vi "Split Registers by Direction.vi"(7 "Group":bool, 8 "error in":errorcluster, 11 "vi info":T1 {"RegisterMap"."Address" format="%.0x"}) -> (0 "error out":errorcluster, 2 "Controls":T8[](array[typedef]) {"Data Type" format="%.0x"}, 3 "Indicator":T8[](array[typedef]) {"Data Type" format="%.0x"})   [LabVIEW 2026, in "FPGA Addon System Explorer.lvlib"]
uses:
  FPGA Addon System Explorer.lvlib
  <userlib>/_OpenG.lib/lvdata/lvdata.llb/openg_variant.lvlib
  Addon Shared/Types/Register Information.ctl
  Addon Shared/FPGA Addon Shared.lvlib
  Submodules/Source/Types/PWM.Measure.Analog.Measurement.ctl
  Submodules/Source/Speciality FPGA IO.lvlib
  Addon Shared/Types/FPGA Addon Data Type.ctl
  Submodules/Source/Types/PWM.Measure.Digital.Measurement.ctl
  Submodules/Source/Types/PWM.Generate.Digital.Settings.ctl
  Submodules/Source/Types/PWM.Measure.Analog.Settings.ctl
  Submodules/Source/Types/PWM.Measure.Digital.Settings.ctl
  Submodules/Source/Types/Sine.Generate.Settings.ctl
  Submodules/Source/Types/Static.Measure.Digital.Measurement.ctl
  Submodules/Source/Types/Static.Generate.Digital.Settings.ctl
  Submodules/Source/Types/Static.Measure.Digital.Settings.ctl
  Submodules/Source/Types/WSS.Generate.Digital.Settings.ctl
  Submodules/Source/Types/QuadratureEncoder.Measure.Digital.Settings.ctl
  Submodules/Source/Types/QuadratureEncoder.Measure.Digital.Measurement.ctl
  <vilib>/fxp/LVFixedPointRepRangeTypeDef.ctl
  <vilib>/fxp/LVFixedPointRepBitsTypeDef.ctl
  <vilib>/Utility/Data Type/NI_Data Type.lvlib
  APIs/FPGA Register IO/TypeDefs/FXP Configuration.ctl
  APIs/FPGA Register IO/FPGA Register IO.lvlib
  <vilib>/picture/picture.llb/imagedata.ctl
  <vilib>/rvi/Bitfile/nirviTypdefDescription.ctl
  <vilib>/rvi/Bitfile/nirviMechanicalAction.ctl
  <vilib>/rvi/Bitfile/nirviClusterElementControl.ctl
  <vilib>/rvi/Bitfile/nirviSubControlStructure.ctl
  <vilib>/rvi/Bitfile/nirviControlStructure.ctl
  <vilib>/rvi/Bitfile/niFpgaBitfileStructure_VI.ctl
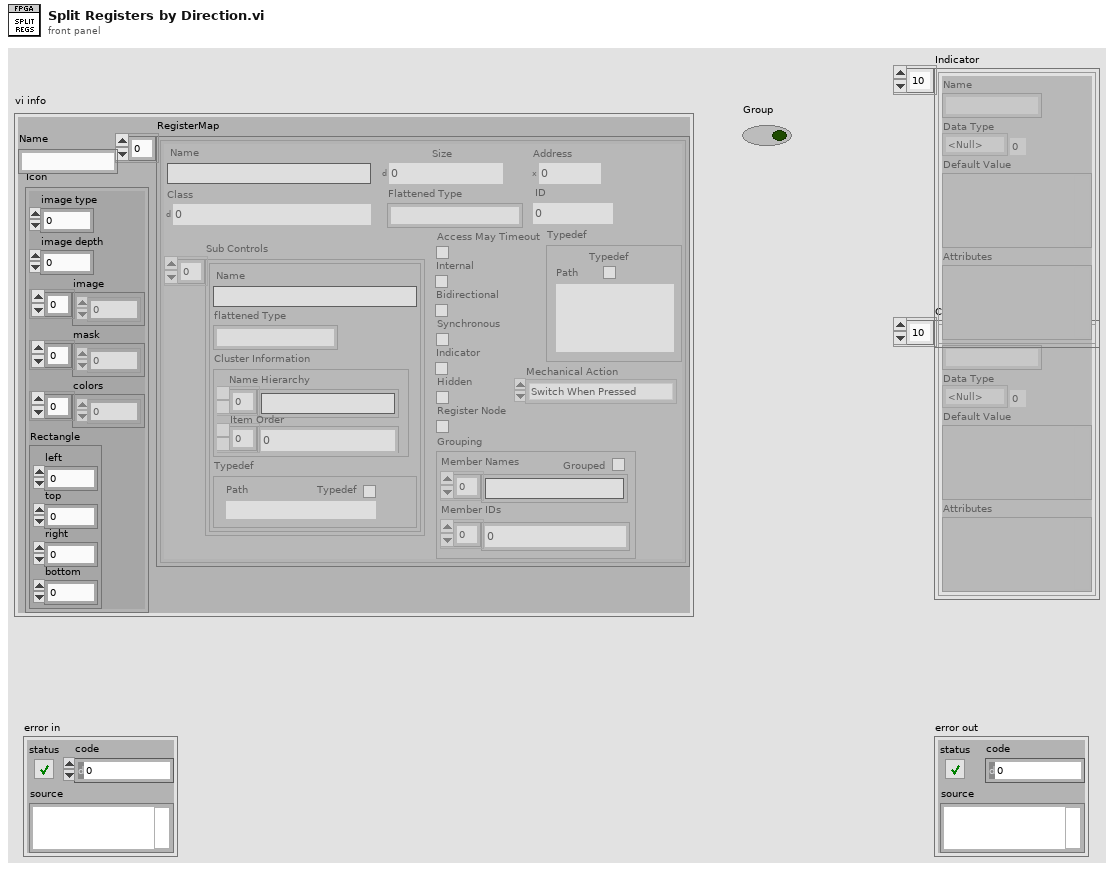
[diagram p1: front panel]
types:
  T1 = typedef "niFpgaBitfileStructure_VI.ctl" = cluster{"Name":string, "RegisterMap":T2[], "Icon":T7}
  T2 = typedef "nirviControlStructure.ctl" = cluster{"Name":string, "Hidden":bool, "Indicator":bool, "Flattened Type":string, "Grouping":cluster{"Grouped":bool, "Member Names":string[], "Member IDs":u32[]}, "Address":u32, "Size":u32, "Class":u32, "Internal":bool, "Typedef":T3, "ID":u32, "Bidirectional":bool, "Synchronous":bool, "Mechanical Action":T4, "Sub Controls":T5[], "Access May Timeout":bool, "Register Node":bool}
  T3 = typedef "nirviTypdefDescription.ctl" = cluster{"Typedef":bool, "Path":path}
  T4 = typedef "nirviMechanicalAction.ctl" = enum8{"Switch When Pressed", "Switch When Released", "Switch Until Released", "Latch When Pressed", "Latch When Released", "Latch Until Released"}
  T5 = typedef "nirviSubControlStructure.ctl" = cluster{"Name":string, "flattened Type":string, "Cluster Information":T6, "Typedef":T3}
  T6 = typedef "nirviClusterElementControl.ctl" = cluster{"Name Hierarchy":string[], "Item Order":u32[]}
  T7 = typedef "imagedata.ctl" = cluster{"image type":i32, "image depth":i32, "image":u8[], "mask":u8[], "colors":u32[], "Rectangle":cluster{"left":i16, "top":i16, "right":i16, "bottom":i16}}
  T8 = typedef "FPGA Addon Shared.lvlib/Register Information.ctl" = cluster{"Name":string, "Data Type":T9, "Default Value":variant, "Attributes":variant}
  T9 = typedef "FPGA Addon Shared.lvlib/FPGA Addon Data Type.ctl" = enum8{"<Null>", "I8", "I16", "I32", "I64", "U8", "U16", "U32", "U64", "SGL", "Boolean", "Analog PWM In Settings", "Analog PWM In", "Digital PWM In Settings", "Digital PWM In", "Digital PWM Out", "Sine Out", "FXP", "FXP+/-24.5", "FXP+/-16.5", "FXP+/-32.8", "FXP+/-64.32", "FXP+/-16.7", "FXP+/-20.5", "FXP+/-27.5", "FXP+/-32.16", "FXP+16.3", "FXP+18.3", "Digital Static In", "Digital Static Out", "Digital Static In Settings", "Digital WSS Out", "Quad Encoder Settings", "Quad Encoder In", "Group"}
  T10 = typedef "Speciality FPGA IO.lvlib/QuadratureEncoder.Measure.Digital.Measurement.ctl" = cluster{"POSITION":i32}
  T11 = typedef "Speciality FPGA IO.lvlib/Static.Measure.Digital.Measurement.ctl" = cluster{"STATE":bool}
  T12 = typedef "Speciality FPGA IO.lvlib/PWM.Measure.Digital.Measurement.ctl" = cluster{"ACTIVE TICKS":u32, "INACTIVE TICKS":u32, "ACQ TICKS":u32}
  T13 = typedef "Speciality FPGA IO.lvlib/PWM.Measure.Analog.Measurement.ctl" = cluster{"ACTIVE TICKS":u32, "INACTIVE TICKS":u32, "ACQ TICKS":u32, "ACTIVE VOLTAGE":fxp<+/-,32,8>, "INACTIVE VOLTAGE":fxp<+/-,32,8>}
  T14 = typedef "Speciality FPGA IO.lvlib/QuadratureEncoder.Measure.Digital.Settings.ctl" = cluster{"DIRECTION":u8, "RESET VALUE":i32, "A RESET STATE":bool, "B RESET STATE":bool, "Z RESET STATE":bool}
  T15 = typedef "Speciality FPGA IO.lvlib/WSS.Generate.Digital.Settings.ctl" = cluster{"ACTIVE EDGE":bool, "ACTIVE TICKS":u32, "INACTIVE TICKS":u32, "DATA":u8, "SENSOR TYPE":u8}
  T16 = typedef "Speciality FPGA IO.lvlib/Static.Measure.Digital.Settings.ctl" = cluster{"ACTIVE EDGE":bool}
  T17 = typedef "Speciality FPGA IO.lvlib/Static.Generate.Digital.Settings.ctl" = cluster{"ACTIVE EDGE":bool, "OUTPUT":bool}
  T18 = typedef "Speciality FPGA IO.lvlib/Sine.Generate.Settings.ctl" = cluster{"AMP":fxp<+/-,32,8>, "OFFSET":fxp<+/-,32,8>, "PERIODS/TICKS":fxp<+,32,0>}
  T19 = typedef "Speciality FPGA IO.lvlib/PWM.Measure.Digital.Settings.ctl" = cluster{"ACTIVE EDGE":bool, "TIMEOUT":u32}
  T20 = typedef "Speciality FPGA IO.lvlib/PWM.Measure.Analog.Settings.ctl" = cluster{"ACTIVE EDGE":bool, "TIMEOUT":u32, "THRESHOLD":fxp<+/-,32,8>}
  T21 = typedef "Speciality FPGA IO.lvlib/PWM.Generate.Digital.Settings.ctl" = cluster{"ACTIVE EDGE":bool, "ACTIVE TICKS":u32, "INACTIVE TICKS":u32}
  T22 = typedef "FPGA Register IO.lvlib/FXP Configuration.ctl" = cluster{"FXP Representation":T23, "FXP Range":T24}
  T23 = typedef "LVFixedPointRepBitsTypeDef.ctl" = cluster{"Signed":bool, "Word Length":u32, "Integer Word Length":i32}
  T24 = typedef "LVFixedPointRepRangeTypeDef.ctl" = cluster{"Range Min":dbl, "Range Max":dbl, "Delta":dbl}
  T25 = typedef "openg_variant.lvlib/Type Descriptor Enumeration__ogtk.ctl" = enum8{"<Null>", "I8", "I16", "I32", "I64", "U8", "U16", "U32", "U64", "SGL", "DBL", "EXT", "CSG", "CDB", "CXT", "0x0F", "0x10", "0x11", "0x12", "0x13", "0x14", "Enum U8", "Enum U16", "Enum U32", "Enum U64", "SGL PQ", "DBL PQ", "EXT PQ", "CSG PQ", "CDB PQ", "CXT PQ", "0x1F", "0x20", "Boolean", "0x22", "0x23", "0x24", "0x25", "0x26", "0x27", "0x28", "0x29", "0x2A", "0x2B", "0x2C", "0x2D", "0x2E", "0x2F", "String", "0x31", "Path", "Pict", "0x34", "0x35", "0x36", "DAQ", "0x38", "0x39", "0x3A", "0x3B", "0x3C", "0x3D", "0x3E", "0x3F", "Array", "0x41", "0x42", "0x43", "0x44", "0x45", "0x46", "0x47", "0x48", "0x49", "0x4A", "0x4B", "0x4C", "0x4D", "0x4E", "0x4F", "Cluster", "0x51", "0x52", "Variant", "Waveform", "0x55", "0x56", "0x57", "0x58", "0x59", "0x5A", "0x5B", "0x5C", "0x5D", "0x5E", "Fixed Point", "0x60", "0x61", "0x62", "0x63", "0x64", "0x65", "0x66", "0x67", "0x68", "0x69", "0x6A", "0x6B", "0x6C", "0x6D", "0x6E", "0x6F", "Refnum", "0x71", "0x72", "Set Collection", "Map Collection"}
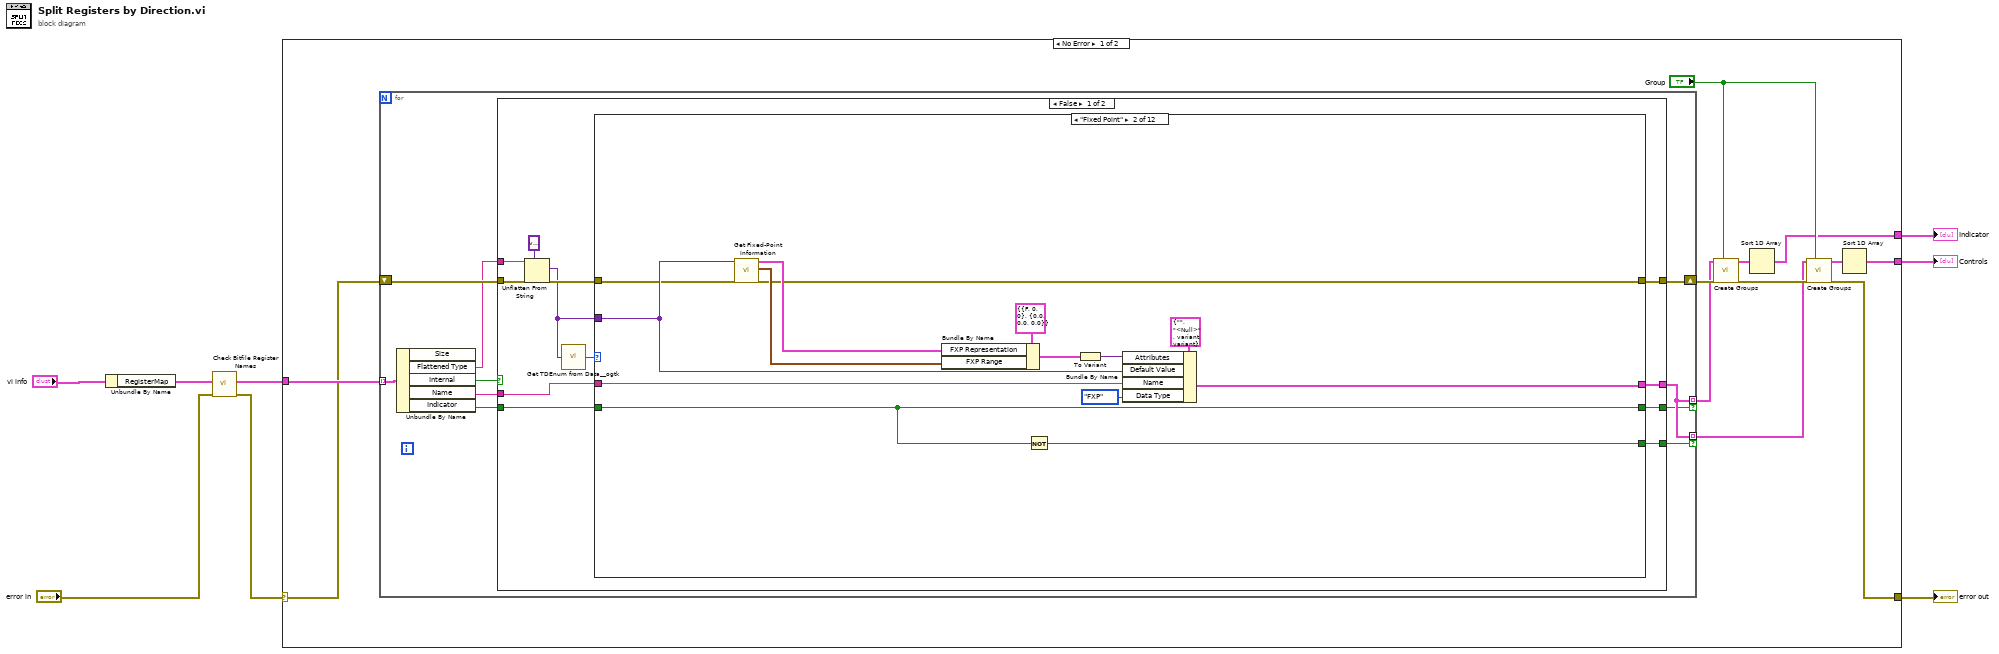
[diagram p0: block diagram]
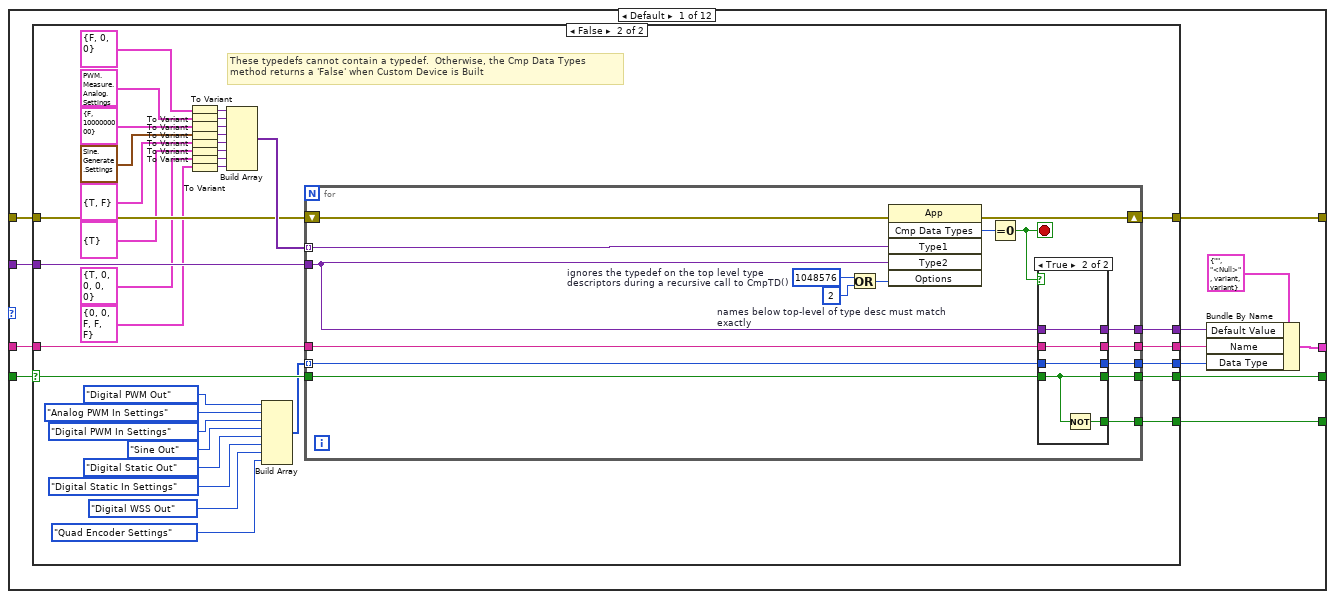
[diagram p2: hidden frame]
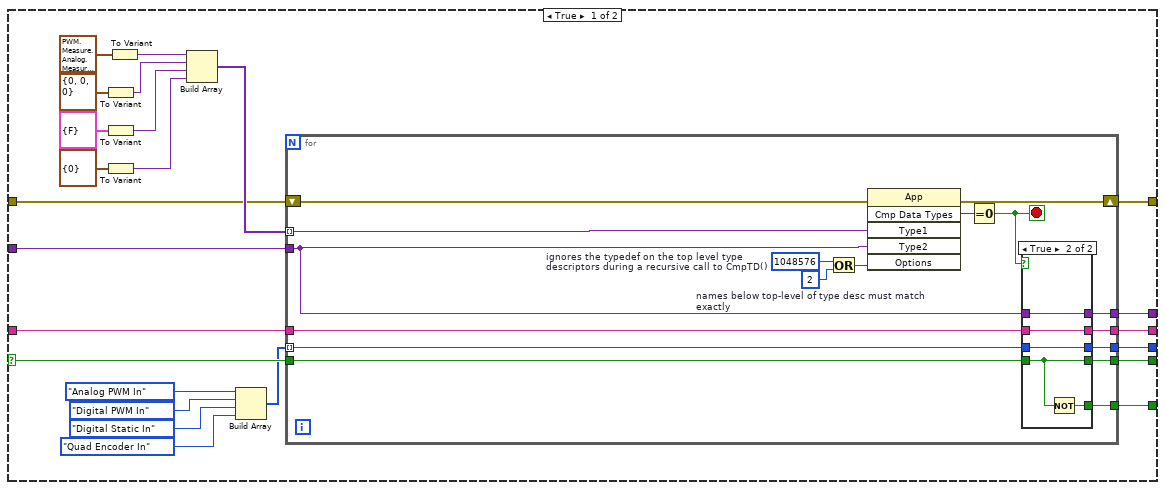
[diagram p3: hidden frame]
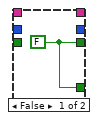
[diagram p4: hidden frame]
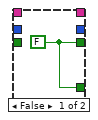
[diagram p5: hidden frame]
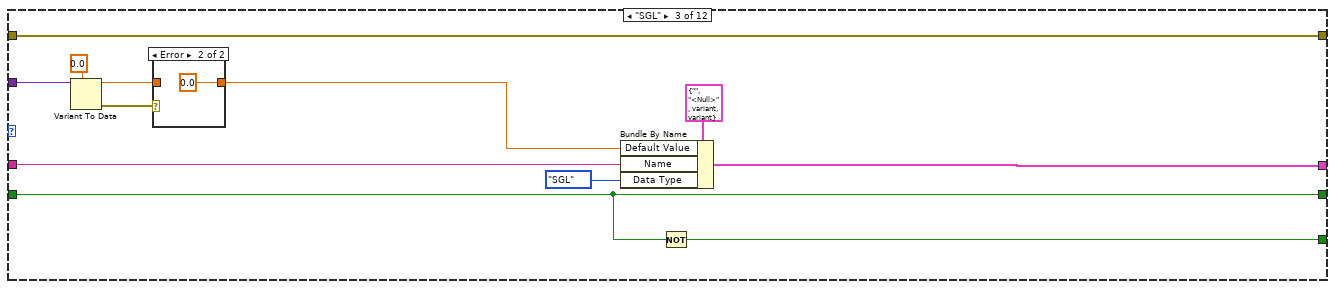
[diagram p6: hidden frame]
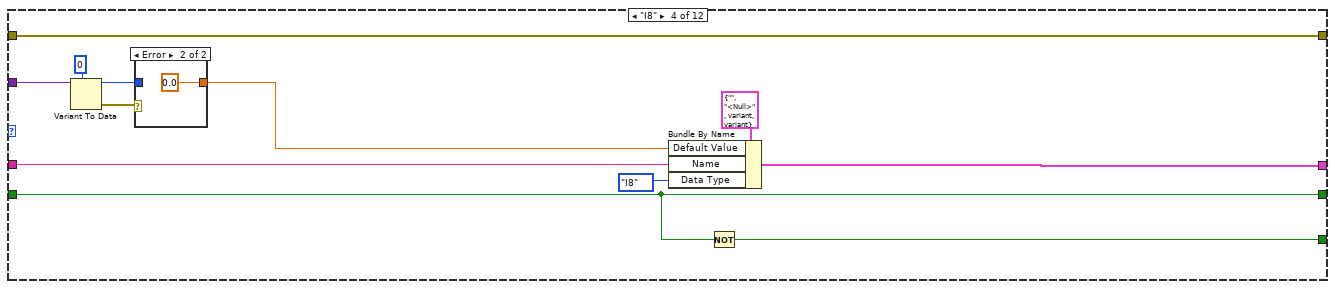
[diagram p8: hidden frame]
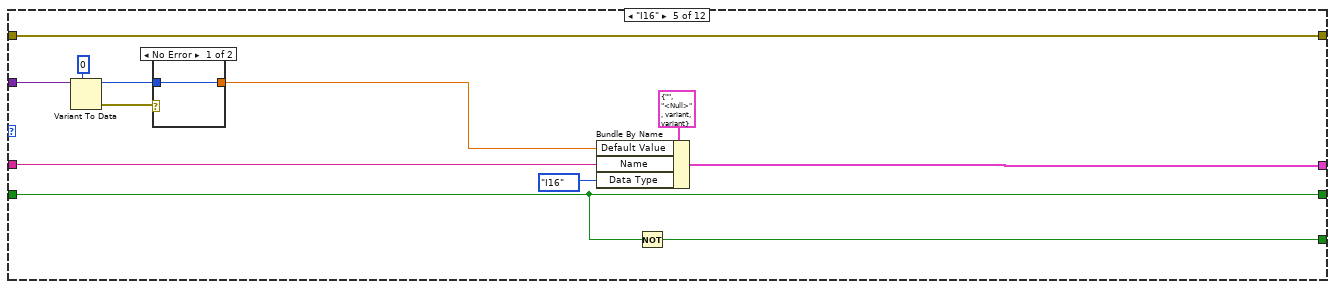
[diagram p10: hidden frame]
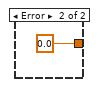
[diagram p11: hidden frame]
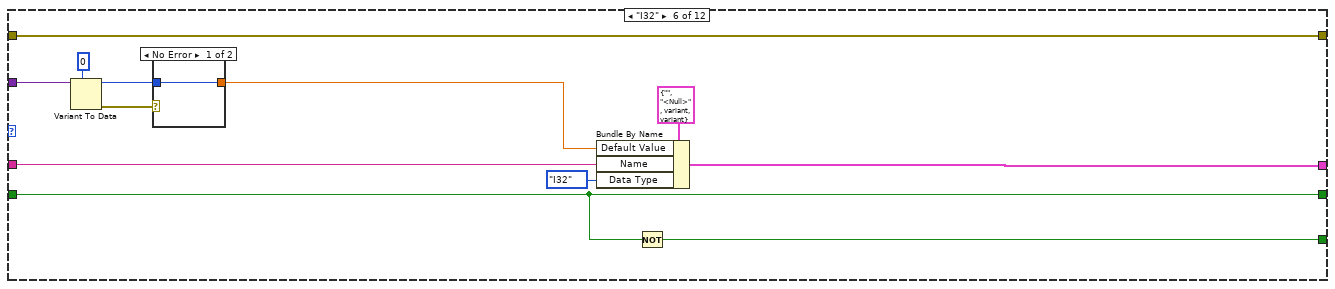
[diagram p12: hidden frame]
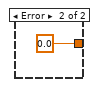
[diagram p13: hidden frame]
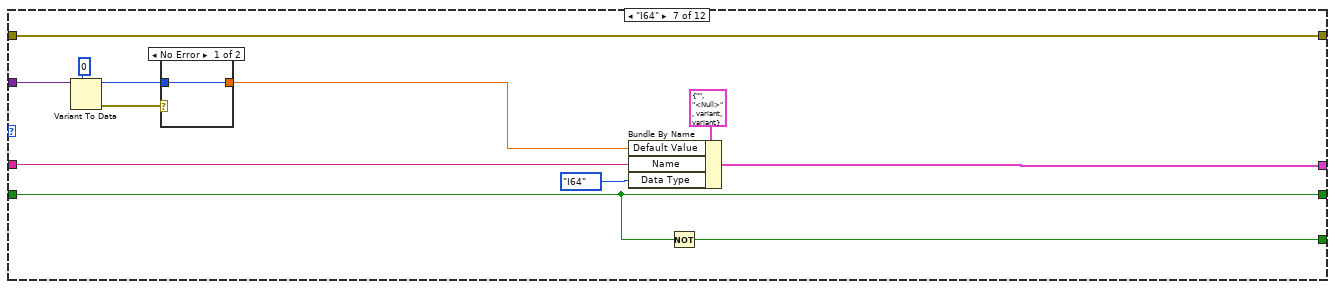
[diagram p14: hidden frame]
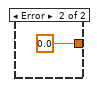
[diagram p15: hidden frame]
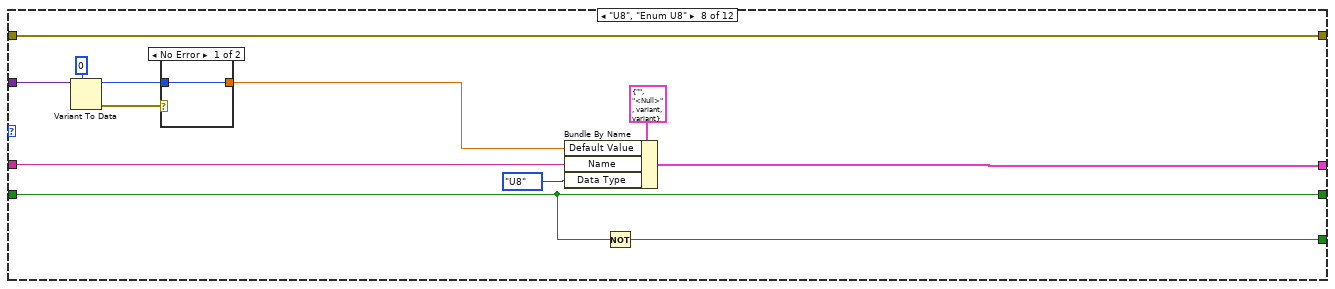
[diagram p16: hidden frame]
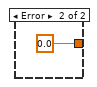
[diagram p17: hidden frame]
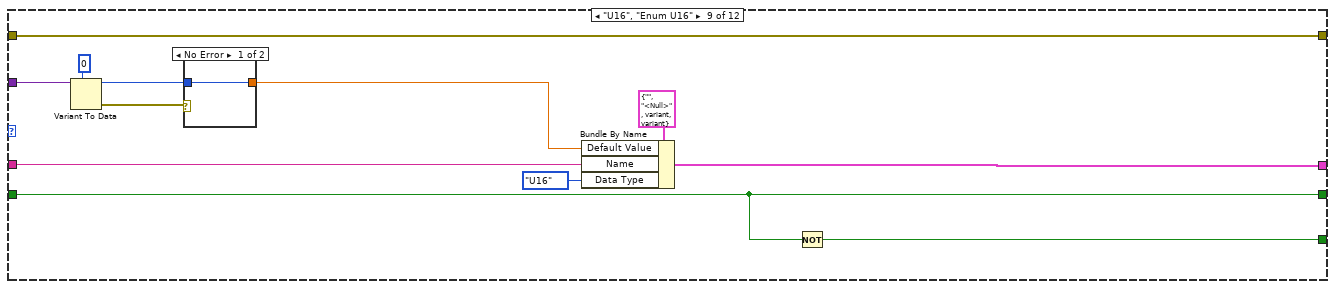
[diagram p18: hidden frame]
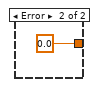
[diagram p19: hidden frame]
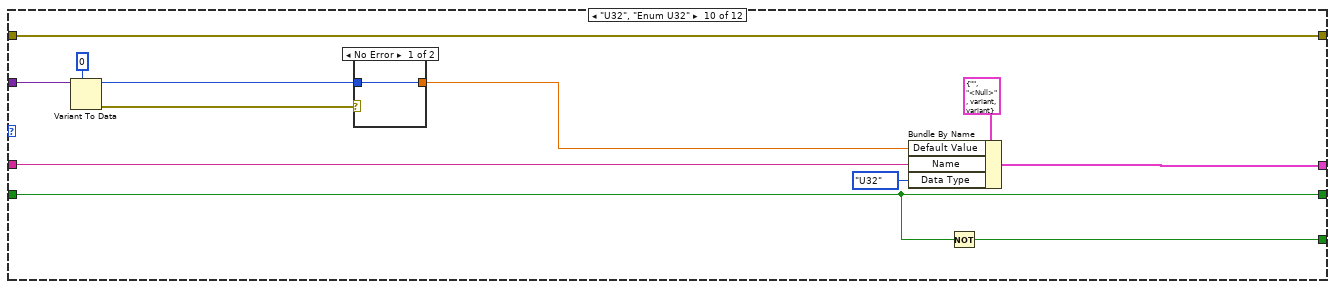
[diagram p20: hidden frame]
diagram:
  n1 = Unbundle By Name("vi info") -> ("RegisterMap"=w4:T2[])
  n2 = call "Check Bitfile Register Names.vi"("error in (no error)"="error in", "RegisterMap in"=w4) -> ("error out"=w1:errorcluster, "RegisterMap out"=w3:T2[])  [unwired: 8 in]
  n3 = case shown="No Error" w1 {
    selector: w1 -> [w9 w318]
    tunnel: [w18 w318] -> w7
    tunnel: [w13 _] -> w6
    tunnel: [w11 _] -> w5
    tunnel: w3 -> [w10 _]
    frame No Error {
      n4 = for {
        tunnel: w10 -> [w25] mode=indexing
        tunnel: [w30] -> w16 mode=indexing if=w29
        tunnel: [w30] -> w15 mode=indexing if=w28
        shift-right: [w27] -> w20
        shift-left: w9 -> [w26]
        n5 = Unbundle By Name(w25) -> ("Flattened Type"=w21:string, "Internal"=w22:bool, "Name"=w23:string, "Indicator"=w24:bool)  [unwired: 1 out]
        n6 = case shown="False" w22 {
          tunnel: w23 -> [w41 _]
          tunnel: w24 -> [w40 _]
          tunnel: [w39 _] -> w30
          tunnel: [w38 w317] -> w29
          tunnel: [w37 w317] -> w28
          tunnel: w21 -> [w34 _]
          tunnel: [w36 w316] -> w27
          tunnel: w26 -> [w33 w316]
          frame False {
            n7 = Unflatten From String(type=variant ("Variant"), binary string=w34, error in (no error)=w33) -> (value=w31:variant, error out=w32:errorcluster)  [unwired: 3 out]
            n8 = call <userlib>:"Get TDEnum from Data__ogtk.vi"("Data"=w31) -> ("Type Descriptor Enumeration"=w42:T25)  [unwired: 4 in]
            n9 = case shown="\"Fixed Point\"" w42 {
              tunnel: [w54 w174 w183 w197 w211 w225 w239 w253 w267 w281 w295 w309] -> w38
              tunnel: w40 -> [w49 w174 w183 w197 w211 w225 w239 w253 w267 w281 w295 w309]
              tunnel: w41 -> [w50 w170 w185 w199 w213 w227 w241 w255 w269 w283 w297 w311]
              tunnel: [w51 w171 w184 w198 w212 w226 w240 w254 w268 w282 w296 w310] -> w39
              tunnel: [w53 w173 w182 w196 w210 w224 w238 w252 w266 w280 w294 w308] -> w37
              tunnel: w31 -> [w48 w168 w181 w195 w209 w223 w237 w251 w265 w279 w293 w307]
              tunnel: [w44 w161 w175 w189 w203 w217 w231 w245 w259 w273 w287 w301] -> w36
              tunnel: w32 -> [w43 w167 w175 w189 w203 w217 w231 w245 w259 w273 w287 w301]
              frame Default {
                n10 = case shown="False" w49 {
                  selector: w49 -> [w73 w133]
                  tunnel: [w78 w137] -> w54
                  tunnel: [w77 w136] -> w53
                  tunnel: w50 -> [w76 w135]
                  tunnel: w48 -> [w67 w129]
                  tunnel: [w66 w128] -> w47
                  tunnel: [w65 w127] -> w46
                  tunnel: [w64 w126] -> w45
                  tunnel: [w62 w117] -> w44
                  tunnel: w43 -> [w61 w118]
                  frame True {
                    n11 = To Variant(anything=T12 {"ACTIVE TICKS"=0, "INACTIVE TICKS"=0, "ACQ TICKS"=0} ("Cached.Data")) -> (Variant=w71:variant)
                    n12 = To Variant(anything=T11 {"STATE"=FALSE} ("Cached.Data")) -> (Variant=w59:variant)
                    n13 = To Variant(anything=T10 {"POSITION"=0} ("Cached.Data")) -> (Variant=w55:variant)
                    n14 = To Variant(anything=T13 {"ACTIVE TICKS"=0, "INACTIVE TICKS"=0, "ACQ TICKS"=0, "ACTIVE VOLTAGE"=0.0, "INACTIVE VOLTAGE"=0.0} ("Cached.Data")) -> (Variant=w72:variant)
                    n15 = Build Array(w72, w71, w59, w55) -> (w68:variant[])
                    n16 = Build Array(FPGA_Addon_Data_Type."Analog PWM In" ("Data Type"), FPGA_Addon_Data_Type."Digital PWM In" ("Data Type"), FPGA_Addon_Data_Type."Digital Static In" ("Data Type"), FPGA_Addon_Data_Type."Quad Encoder In" ("Data Type")) -> (w63:T9[])
                    n17 = for {
                      tunnel: w67 -> [w82]
                      tunnel: [w93] -> w77
                      tunnel: w76 -> [w92]
                      tunnel: w68 -> [w84] mode=indexing
                      tunnel: [w91] -> w65
                      tunnel: [w90] -> w66
                      tunnel: [w89] -> w64
                      tunnel: w63 -> [w88] mode=indexing
                      tunnel: w73 -> [w95]
                      tunnel: [w94] -> w78
                      shift-right: [w79] -> w62
                      shift-left: w61 -> [w80]
                      stop <- w83 stop-if-true
                      w81 = 2  # names below top-level of type desc must match exactly
                      w86 = 1048576  # ignores the typedef on the top level type descriptors during a recursive call to CmpTD()
                      n18 = Or(x=w86, y=w81) -> (x .or. y?=w87:i32)
                      n19 = invoke class="App" method="Cmp Data Types"(error in=w80, "Type1"=w84, "Type2"=w82, "Options"=w87) -> (error out=w79:errorcluster, "Compare Data Types"=w85:i32)  [unwired: 2 in, 4 out]
                      n20 = Equal To 0?(x=w85) -> (x = 0?=w83:bool)
                      n21 = case shown="True" w83 {
                        tunnel: w95 -> [_ w101]
                        tunnel: [w96 w101] -> w94
                        tunnel: [w96 w100] -> w93
                        tunnel: w92 -> [_ w98]
                        tunnel: [_ w99] -> w91
                        tunnel: w82 -> [_ w99]
                        tunnel: [_ w98] -> w90
                        tunnel: [_ w97] -> w89
                        tunnel: w88 -> [_ w97]
                        frame False {
                          w96 = FALSE ("Boolean")
                        }
                        frame True {
                          n22 = Not(x=w101) -> (.not. x?=w100:bool)
                        }
                      }
                    }
                  }
                  frame False {
                    # "These typedefs cannot contain a typedef.  Otherwise, the Cmp Data Types \nmethod returns a 'False' when Custom Device is Built"
                    n23 = To Variant(anything=T21 {"ACTIVE EDGE"=FALSE, "ACTIVE TICKS"=0, "INACTIVE TICKS"=0} ("Channel.Settings")) -> (Variant=w132:variant)
                    n24 = To Variant(anything=T20 {"ACTIVE EDGE"=FALSE, "TIMEOUT"=1000000000, "THRESHOLD"=3.0} ("Channel.Settings")) -> (Variant=w122:variant)
                    n25 = To Variant(anything=T19 {"ACTIVE EDGE"=FALSE, "TIMEOUT"=1000000000} ("Channel.Settings")) -> (Variant=w121:variant)
                    n26 = To Variant(anything=T18 {"AMP"=0.0, "OFFSET"=0.0, "PERIODS/TICKS"=0.0002500000409781933} ("Settings")) -> (Variant=w115:variant)
                    n27 = To Variant(anything=T17 {"ACTIVE EDGE"=TRUE, "OUTPUT"=FALSE} ("Settings")) -> (Variant=w113:variant)
                    n28 = To Variant(anything=T16 {"ACTIVE EDGE"=TRUE} ("Settings")) -> (Variant=w110:variant)
                    n29 = To Variant(anything=T15 {"ACTIVE EDGE"=TRUE, "ACTIVE TICKS"=0, "INACTIVE TICKS"=0, "DATA"=0, "SENSOR TYPE"=0} ("Wheel Speed Sensor Settings")) -> (Variant=w106:variant)
                    n30 = To Variant(anything=T14 {"DIRECTION"=0, "RESET VALUE"=0, "A RESET STATE"=FALSE, "B RESET STATE"=FALSE, "Z RESET STATE"=FALSE} ("Settings")) -> (Variant=w103:variant)
                    n31 = Build Array(w132, w122, w121, w115, w113, w110, w106, w103) -> (w130:variant[])
                    n32 = Build Array(FPGA_Addon_Data_Type."Digital PWM Out" ("Data Type"), FPGA_Addon_Data_Type."Analog PWM In Settings" ("Data Type"), FPGA_Addon_Data_Type."Digital PWM In Settings" ("Data Type"), FPGA_Addon_Data_Type."Sine Out" ("Data Type"), FPGA_Addon_Data_Type."Digital Static Out" ("Data Type"), FPGA_Addon_Data_Type."Digital Static In Settings" ("Data Type"), FPGA_Addon_Data_Type."Digital WSS Out" ("Data Type"), FPGA_Addon_Data_Type."Quad Encoder Settings" ("Data Type")) -> (w125:T9[])
                    n33 = for {
                      tunnel: w129 -> [w143]
                      tunnel: [w152] -> w136
                      tunnel: w135 -> [w151]
                      tunnel: w130 -> [w142] mode=indexing
                      tunnel: [w150] -> w127
                      tunnel: [w149] -> w128
                      tunnel: [w148] -> w126
                      tunnel: w125 -> [w147] mode=indexing
                      tunnel: w133 -> [w154]
                      tunnel: [w153] -> w137
                      shift-right: [w138] -> w117
                      shift-left: w118 -> [w139]
                      stop <- w140 stop-if-true
                      w145 = 2  # names below top-level of type desc must match exactly
                      w144 = 1048576  # ignores the typedef on the top level type descriptors during a recursive call to CmpTD()
                      n34 = Or(x=w144, y=w145) -> (x .or. y?=w146:i32)
                      n35 = invoke class="App" method="Cmp Data Types"(error in=w139, "Type1"=w142, "Type2"=w143, "Options"=w146) -> (error out=w138:errorcluster, "Compare Data Types"=w141:i32)  [unwired: 2 in, 4 out]
                      n36 = Equal To 0?(x=w141) -> (x = 0?=w140:bool)
                      n37 = case shown="True" w140 {
                        tunnel: w154 -> [_ w160]
                        tunnel: [w155 w160] -> w153
                        tunnel: [w155 w159] -> w152
                        tunnel: w151 -> [_ w157]
                        tunnel: [_ w158] -> w150
                        tunnel: w143 -> [_ w158]
                        tunnel: [_ w157] -> w149
                        tunnel: [_ w156] -> w148
                        tunnel: w147 -> [_ w156]
                        frame False {
                          w155 = FALSE ("Boolean")
                        }
                        frame True {
                          n38 = Not(x=w160) -> (.not. x?=w159:bool)
                        }
                      }
                    }
                  }
                }
                n39 = Bundle By Name(cluster=T8 {"Name"="", "Data Type"=enum."<Null>", "Default Value"=variant(refnum<class> refnum), "Attributes"=variant}, "Default Value"=w46, "Name"=w47, "Data Type"=w45) -> (w51:T8)
              }
              frame "Fixed Point" {
                n40 = call <vilib>:"Get Fixed-Point Information.vi"("error in (no error)"=w167, "variant"=w168) -> ("error out"=w161:errorcluster, "FXP range"=w164:T24, "FXP representation"=w165:T23)  [unwired: 6 in, 1 out]
                n41 = Bundle By Name(cluster=T22 {"FXP Representation"={"Signed"=FALSE, "Word Length"=0, "Integer Word Length"=0}, "FXP Range"={"Range Min"=0.0, "Range Max"=0.0, "Delta"=0.0}} ("FXP Configuration"), "FXP Representation"=w165, "FXP Range"=w164) -> (w163:T22)
                n42 = Not(x=w174) -> (.not. x?=w173:bool)
                n43 = To Variant(anything=w163) -> (Variant=w162:variant)
                n44 = Bundle By Name(cluster=T8 {"Name"="", "Data Type"=enum."<Null>", "Default Value"=variant(refnum<class> refnum), "Attributes"=variant}, "Attributes"=w162, "Default Value"=w168, "Name"=w170, "Data Type"=FPGA_Addon_Data_Type."FXP") -> (w171:T8)
              }
              frame "SGL" {
                n45 = Variant To Data(type=sgl 0.0, Variant=w181) -> (data=w177:sgl, error out=w179:errorcluster)  [unwired: 1 in]
                n46 = case shown="Error" w179 {
                  tunnel: [w187 0.0] -> w178
                  tunnel: w177 -> [w187 _]
                  frame No Error {
                  }
                  frame Error {
                  }
                }
                n47 = Bundle By Name(cluster=T8 {"Name"="", "Data Type"=enum."<Null>", "Default Value"=variant(refnum<class> refnum), "Attributes"=variant}, "Default Value"=w178, "Name"=w185, "Data Type"=FPGA_Addon_Data_Type."SGL") -> (w184:T8)
                n48 = Not(x=w183) -> (.not. x?=w182:bool)
              }
              frame "I8" {
                n49 = Variant To Data(type=i8 0, Variant=w195) -> (data=w191:i8, error out=w193:errorcluster)  [unwired: 1 in]
                n50 = case shown="Error" w193 {
                  tunnel: [w201 0.0] -> w192
                  tunnel: w191 -> [w201 _]
                  frame No Error {
                  }
                  frame Error {
                  }
                }
                n51 = Bundle By Name(cluster=T8 {"Name"="", "Data Type"=enum."<Null>", "Default Value"=variant(refnum<class> refnum), "Attributes"=variant}, "Default Value"=w192, "Name"=w199, "Data Type"=FPGA_Addon_Data_Type."I8") -> (w198:T8)
                n52 = Not(x=w197) -> (.not. x?=w196:bool)
              }
              frame "I16" {
                n53 = Variant To Data(type=i16 0, Variant=w209) -> (data=w205:i16, error out=w207:errorcluster)  [unwired: 1 in]
                n54 = case shown="No Error" w207 {
                  tunnel: [w215 0.0] -> w206
                  tunnel: w205 -> [w215 _]
                  frame No Error {
                  }
                  frame Error {
                  }
                }
                n55 = Bundle By Name(cluster=T8 {"Name"="", "Data Type"=enum."<Null>", "Default Value"=variant(refnum<class> refnum), "Attributes"=variant}, "Default Value"=w206, "Name"=w213, "Data Type"=FPGA_Addon_Data_Type."I16") -> (w212:T8)
                n56 = Not(x=w211) -> (.not. x?=w210:bool)
              }
              frame "I32" {
                n57 = Variant To Data(type=0, Variant=w223) -> (data=w219:i32, error out=w221:errorcluster)  [unwired: 1 in]
                n58 = case shown="No Error" w221 {
                  tunnel: [w229 0.0] -> w220
                  tunnel: w219 -> [w229 _]
                  frame No Error {
                  }
                  frame Error {
                  }
                }
                n59 = Bundle By Name(cluster=T8 {"Name"="", "Data Type"=enum."<Null>", "Default Value"=variant(refnum<class> refnum), "Attributes"=variant}, "Default Value"=w220, "Name"=w227, "Data Type"=FPGA_Addon_Data_Type."I32") -> (w226:T8)
                n60 = Not(x=w225) -> (.not. x?=w224:bool)
              }
              frame "I64" {
                n61 = Variant To Data(type=i64 0, Variant=w237) -> (data=w233:i64, error out=w235:errorcluster)  [unwired: 1 in]
                n62 = case shown="No Error" w235 {
                  tunnel: [w243 0.0] -> w234
                  tunnel: w233 -> [w243 _]
                  frame No Error {
                  }
                  frame Error {
                  }
                }
                n63 = Bundle By Name(cluster=T8 {"Name"="", "Data Type"=enum."<Null>", "Default Value"=variant(refnum<class> refnum), "Attributes"=variant}, "Default Value"=w234, "Name"=w241, "Data Type"=FPGA_Addon_Data_Type."I64") -> (w240:T8)
                n64 = Not(x=w239) -> (.not. x?=w238:bool)
              }
              frame "U8", "Enum U8" {
                n65 = Variant To Data(type=u8 0, Variant=w251) -> (data=w247:u8, error out=w249:errorcluster)  [unwired: 1 in]
                n66 = case shown="No Error" w249 {
                  tunnel: [w257 0.0] -> w248
                  tunnel: w247 -> [w257 _]
                  frame No Error {
                  }
                  frame Error {
                  }
                }
                n67 = Bundle By Name(cluster=T8 {"Name"="", "Data Type"=enum."<Null>", "Default Value"=variant(refnum<class> refnum), "Attributes"=variant}, "Default Value"=w248, "Name"=w255, "Data Type"=FPGA_Addon_Data_Type."U8") -> (w254:T8)
                n68 = Not(x=w253) -> (.not. x?=w252:bool)
              }
              frame "U16", "Enum U16" {
                n69 = Variant To Data(type=u16 0, Variant=w265) -> (data=w261:u16, error out=w263:errorcluster)  [unwired: 1 in]
                n70 = case shown="No Error" w263 {
                  tunnel: [w271 0.0] -> w262
                  tunnel: w261 -> [w271 _]
                  frame No Error {
                  }
                  frame Error {
                  }
                }
                n71 = Bundle By Name(cluster=T8 {"Name"="", "Data Type"=enum."<Null>", "Default Value"=variant(refnum<class> refnum), "Attributes"=variant}, "Default Value"=w262, "Name"=w269, "Data Type"=FPGA_Addon_Data_Type."U16") -> (w268:T8)
                n72 = Not(x=w267) -> (.not. x?=w266:bool)
              }
              frame "U32", "Enum U32" {
                n73 = Variant To Data(type=u32 0, Variant=w279) -> (data=w275:u32, error out=w277:errorcluster)  [unwired: 1 in]
                n74 = case shown="No Error" w277 {
                  tunnel: [w285 0.0] -> w276
                  tunnel: w275 -> [w285 _]
                  frame No Error {
                  }
                  frame Error {
                  }
                }
                n75 = Bundle By Name(cluster=T8 {"Name"="", "Data Type"=enum."<Null>", "Default Value"=variant(refnum<class> refnum), "Attributes"=variant}, "Default Value"=w276, "Name"=w283, "Data Type"=FPGA_Addon_Data_Type."U32") -> (w282:T8)
                n76 = Not(x=w281) -> (.not. x?=w280:bool)
              }
              frame "U64", "Enum U64" {
                n77 = Variant To Data(type=u64 0, Variant=w293) -> (data=w289:u64, error out=w291:errorcluster)  [unwired: 1 in]
                n78 = case shown="No Error" w291 {
                  tunnel: [w299 0.0] -> w290
                  tunnel: w289 -> [w299 _]
                  frame No Error {
                  }
                  frame Error {
                  }
                }
                n79 = Bundle By Name(cluster=T8 {"Name"="", "Data Type"=enum."<Null>", "Default Value"=variant(refnum<class> refnum), "Attributes"=variant}, "Default Value"=w290, "Name"=w297, "Data Type"=FPGA_Addon_Data_Type."U64") -> (w296:T8)
                n80 = Not(x=w295) -> (.not. x?=w294:bool)
              }
              frame "Boolean" {
                n81 = Variant To Data(type=FALSE, Variant=w307) -> (data=w303:bool, error out=w305:errorcluster)  [unwired: 1 in]
                n82 = case shown="No Error" w305 {
                  tunnel: [w313 0.0] -> w304
                  tunnel: w303 -> [w314 _]
                  frame No Error {
                    n83 = Boolean To (0,1)(Boolean=w314) -> (0, 1=w313:i16)
                  }
                  frame Error {
                  }
                }
                n84 = Bundle By Name(cluster=T8 {"Name"="", "Data Type"=enum."<Null>", "Default Value"=variant(refnum<class> refnum), "Attributes"=variant}, "Default Value"=w304, "Name"=w311, "Data Type"=FPGA_Addon_Data_Type."Boolean") -> (w310:T8)
                n85 = Not(x=w309) -> (.not. x?=w308:bool)
              }
            }
          }
          frame True {
            w317 = FALSE ("Boolean")
          }
        }
      }
      n86 = call "Create Groups.vi"("Group"="Group", "error in (no error)"=w20, "Channels"=w16) -> ("error out"=w19:errorcluster, "Channels out"=w14:T8[])  [unwired: 7 in]
      n87 = Sort 1D Array(array=w14) -> (sorted array=w13:T8[])
      n88 = call "Create Groups.vi"("Group"="Group", "error in (no error)"=w19, "Channels"=w15) -> ("error out"=w18:errorcluster, "Channels out"=w12:T8[])  [unwired: 7 in]
      n89 = Sort 1D Array(array=w12) -> (sorted array=w11:T8[])
    }
    frame Error {
    }
  }
  "Controls" <- w5
  "Indicator" <- w6
  "error out" <- w7
